vi "BRig_dataLC_Wrong_Delay_l1.vi"() -> (2 "output_Wrong_Delay":i32)   [LabVIEW 2014]
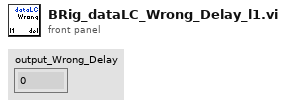
[diagram p1: front panel]
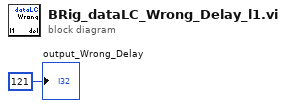
[diagram p0: block diagram]
diagram:
  "output_Wrong_Delay" <- 121 ("output_iBlock")
